vi "RTK-Make window child of calling VI.vi"(4 "Scrollbars (No change)":i32(ring)=2 items=["Hide", "Show", "No change"], 5 "Window Number (0...22)":i32 min=0 max=22, 6 "error in (no error)":errorcluster, 7 "Name of Parent Panel":string, 8 "Width & Height":cluster{"Width":u32, "Height":u32}, 9 "Coordinates (panel)":cluster{"Left":i32, "Top":i32}={"Left"=40, "Top"=40}) -> (0 "error out":errorcluster)   [LabVIEW 2018]
doc: "Developer: Wayne Lootsma\nDate: 12/30/2002\nDescription:\nMake the IMAQ window a child of the specified vi.\n\nDialog Panel: False\nGUI Panel: False"
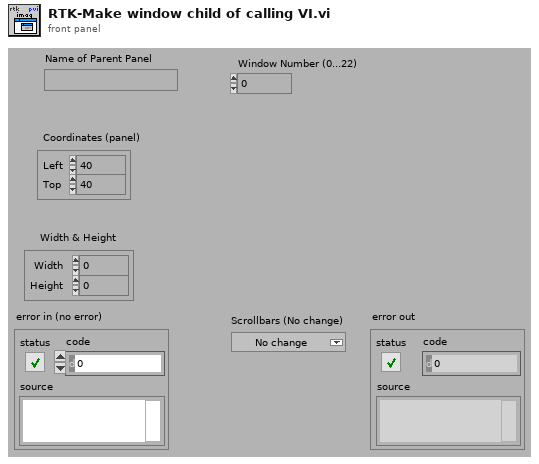
[diagram p1: front panel]
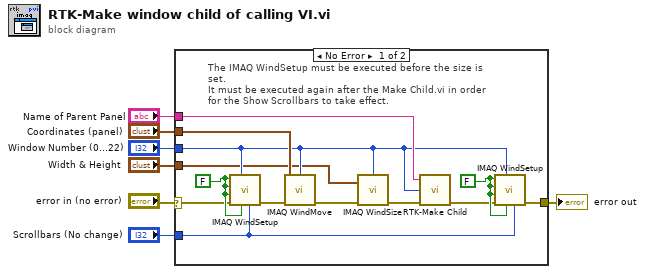
[diagram p0: block diagram]
diagram:
  n1 = case shown="No Error" "error in (no error)" {
    selector: "error in (no error)" -> [w9 w21]
    tunnel: "Coordinates (panel)" -> [w18 _]
    tunnel: "Name of Parent Panel" -> [w17 _]
    tunnel: [w14 w21] -> w5
    tunnel: "Scrollbars (No change)" -> [w11 _]
    tunnel: "Window Number (0...22)" -> [w10 _]
    tunnel: "Width & Height" -> [w8 _]
    frame No Error {
      w13 = FALSE ("Window can grow? (Yes)")
      w16 = FALSE ("Window can grow? (Yes)")
      # "The IMAQ WindSetup must be executed before the size is set.\nIt must be executed again after the Make Child.vi in order for the Show Scrollbars to take effect."
      n2 = call "IMAQ WindSetup"("Scrollbars (No change)"=w11, "Window is floating? (No)"=w13, "Window Number (0...15)"=w10, "error in (no error)"=w9, "Window has title bar? (Yes)"=w13, "Window can close? (Yes)"=w13, "Window can grow? (Yes)"=w13) -> ("error out"=w12:errorcluster)  [unwired: 4 in]
      n3 = call "IMAQ WindMove"("Window Number (0...15)"=w10, "Coordinates (screen)"=w18, "error in (no error)"=w12) -> ("error out"=w20:errorcluster)  [unwired: 2 in, 1 out]
      n4 = call "IMAQ WindSize"("error in (no error)"=w20, "Width & Height"=w8, "Window Number"=w10) -> ("error out"=w19:errorcluster)  [unwired: 3 in, 2 out]
      n5 = call "RTK-Make Child.vi"("error in (no error)"=w19, "Window Number"=w10, "Name of Parent Panel"=w17) -> ("error out"=w15:errorcluster)
      n6 = call "IMAQ WindSetup"("Scrollbars (No change)"=w11, "Window is floating? (No)"=w16, "Window Number (0...15)"=w10, "error in (no error)"=w15, "Window has title bar? (Yes)"=w16, "Window can close? (Yes)"=w16, "Window can grow? (Yes)"=w16) -> ("error out"=w14:errorcluster)  [unwired: 4 in]
    }
    frame Error {
    }
  }
  "error out" <- w5
